vi "canDataSort.vi"() -> ()   [LabVIEW 2023] (continued)
16\t39\t88\r\n      2202  1FFFFFFF   00000004    8        00\t00\tFF\tFF\tFF\tFF\tFF\tFF\r\n      2193  18F106A7   00000004    8        00\tF7\tFF\tFF\tFF\tFF\tFF\t9C\r\n      2192  1FFFFFFF   00000004    8        00\t00\tFF\tFF\tFF\tFF\tFF\tFF\r\n      2183  0CF102A7   00000004    8        30\t75\tE0\t2E\t80\tFF\tFF\tFD\r\n      2183  0CF101A7   00000004    8        68\t00\t97\tCC\t00\t16\t39\t87\r\n      2182  1FFFFFFF   00000004    8        00\t00\tFF\tFF\tFF\tFF\tFF\tFF\r\n      2172  1FFFFFFF   00000004    8        00\t00\tFF\tFF\tFF\tFF\tFF\tFF\r\n      2223  0CF101A7   00000004    8        68\t00\t97\tCC\t00\t16\t39\t89\r\n      2222  1FFFFFFF   00000004    8        00\t00\tFF\tFF\tFF\tFF\tFF\tFF\r\n      2212  1FFFFFFF   00000004    8        00\t20\tFF\tFF\tFF\tFF\tFF\tFF\r\n      2203  0CF102A7   00000004    8        30\t75\tE0\t2E\t80\tFF\tFF\tFD\r\n      2203  0CF101A7   00000004    8        68\t00\t97\tCC\t00\t16\t39\t88\r\n      2202  1FFFFFFF   00000004    8        00\t00\tFF\tFF\tFF\tFF\tFF\tFF\r\n      2193  18F106A7   00000004    8        00\tF7\tFF\tFF\tFF\tFF\tFF\t9C\r\n      2192  1FFFFFFF   00000004    8        00\t00\tFF\tFF\tFF\tFF\tFF\tFF\r\n      2183  0CF102A7   00000004    8        30\t75\tE0\t2E\t80\tFF\tFF\tFD\r\n      2183  0CF101A7   00000004    8        68\t00\t97\tCC\t00\t16\t39\t87\r\n      2182  1FFFFFFF   00000004    8        00\t00\tFF\tFF\tFF\tFF\tFF\tFF\r\n      2223  0CF102A7   00000004    8        30\t75\tE0\t2E\t80\tFF\tFF\tFD\r\n      2223  0CF101A7   00000004    8        68\t00\t97\tCC\t00\t16\t39\t89\r\n      2222  1FFFFFFF   00000004    8        00\t00\tFF\tFF\tFF\tFF\tFF\tFF\r\n      2212  1FFFFFFF   00000004    8        00\t20\tFF\tFF\tFF\tFF\tFF\tFF\r\n      2203  0CF102A7   00000004    8        30\t75\tE0\t2E\t80\tFF\tFF\tFD\r\n      2203  0CF101A7   00000004    8        68\t00\t97\tCC\t00\t16\t39\t88\r\n      2202  1FFFFFFF   00000004    8        00\t00\tFF\tFF\tFF\tFF\tFF\tFF\r\n      2193  18F106A7   00000004    8        00\tF7\tFF\tFF\tFF\tFF\tFF\t9C\r\n      2192  1FFFFFFF   00000004    8        00\t00\tFF\tFF\tFF\tFF\tFF\tFF\r\n      2183  0CF102A7   00000004    8        30\t75\tE0\t2E\t80\tFF\tFF\tFD\r\n      2183  0CF101A7   00000004    8        68\t00\t97\tCC\t00\t16\t39\t87\r\n      2232  1FFFFFFF   00000004    8        00\t00\tFF\tFF\tFF\tFF\tFF\tFF\r\n      2223  0CF102A7   00000004    8        30\t75\tE0\t2E\t80\tFF\tFF\tFD\r\n      2223  0CF101A7   00000004    8        68\t00\t97\tCC\t00\t16\t39\t89\r\n      2222  1FFFFFFF   00000004    8        00\t00\tFF\tFF\tFF\tFF\tFF\tFF\r\n      2212  1FFFFFFF   00000004    8        00\t20\tFF\tFF\tFF\tFF\tFF\tFF\r\n      2203  0CF102A7   00000004    8        30\t75\tE0\t2E\t80\tFF\tFF\tFD\r\n      2203  0CF101A7   00000004    8        68\t00\t97\tCC\t00\t16\t39\t88\r\n      2202  1FFFFFFF   00000004    8        00\t00\tFF\tFF\tFF\tFF\tFF\tFF\r\n      2193  18F106A7   00000004    8        00\tF7\tFF\tFF\tFF\tFF\tFF\t9C\r\n      2192  1FFFFFFF   00000004    8        00\t00\tFF\tFF\tFF\tFF\tFF\tFF\r\n      2183  0CF102A7   00000004    8        30\t75\tE0\t2E\t80\tFF\tFF\tFD\r\n      2241  18F11FF0   00000004    8        FF\t3F\t90\t68\t88\t1B\t10\tEC\r\n      2232  1FFFFFFF   00000004    8        00\t00\tFF\tFF\tFF\tFF\tFF\tFF\r\n      2223  0CF102A7   00000004    8        30\t75\tE0\t2E\t80\tFF\tFF\tFD\r\n      2223  0CF101A7   00000004    8        68\t00\t97\tCC\t00\t16\t39\t89\r\n      2222  1FFFFFFF   00000004    8        00\t00\tFF\tFF\tFF\tFF\tFF\tFF\r\n      2212  1FFFFFFF   00000004    8        00\t20\tFF\tFF\tFF\tFF\tFF\tFF\r\n      2203  0CF102A7   00000004    8        30\t75\tE0\t2E\t80\tFF\tFF\tFD\r\n      2203  0CF101A7   00000004    8        68\t00\t97\tCC\t00\t16\t39\t88\r\n      2202  1FFFFFFF   00000004    8        00\t00\tFF\tFF\tFF\tFF\tFF\tFF\r\n      2193  18F106A7   00000004    8        00\tF7\tFF\tFF\tFF\tFF\tFF\t9C\r\n      2192  1FFFFFFF   00000004    8        00\t00\tFF\tFF\tFF\tFF\tFF\tFF\r\n      2242  18F120F0   00000004    8        2B\t75\t60\tB1\tB0\t01\tFF\tFF\r\n      2241  18F11FF0   00000004    8        FF\t3F\t90\t68\t88\t1B\t10\tEC\r\n      2232  1FFFFFFF   00000004    8        00\t00\tFF\tFF\tFF\tFF\tFF\tFF\r\n      2223  0CF102A7   00000004    8        30\t75\tE0\t2E\t80\tFF\tFF\tFD\r\n      2223  0CF101A7   00000004    8        68\t00\t97\tCC\t00\t16\t39\t89\r\n      2222  1FFFFFFF   00000004    8        00\t00\tFF\tFF\tFF\tFF\tFF\tFF\r\n      2212  1FFFFFFF   00000004    8        00\t20\tFF\tFF\tFF\tFF\tFF\tFF\r\n      2203  0CF102A7   00000004    8        30\t75\tE0\t2E\t80\tFF\tFF\tFD\r\n      2203  0CF101A7   00000004    8        68\t00\t97\tCC\t00\t16\t39\t88\r\n      2202  1FFFFFFF   00000004    8        00\t00\tFF\tFF\tFF\tFF\tFF\tFF\r\n      2193  18F106A7   00000004    8        00\tF7\tFF\tFF\tFF\tFF\tFF\t9C\r\n      2243  0CF101A7   00000004    8        68\t00\t97\tCC\t00\t16\t39\t8A\r\n      2242  18F120F0   00000004    8        2B\t75\t60\tB1\tB0\t01\tFF\tFF\r\n      2241  18F11FF0   00000004    8        FF\t3F\t90\t68\t88\t1B\t10\tEC\r\n      2232  1FFFFFFF   00000004    8        00\t00\tFF\tFF\tFF\tFF\tFF\tFF\r\n      2223  0CF102A7   00000004    8        30\t75\tE0\t2E\t80\tFF\tFF\tFD\r\n      2223  0CF101A7   00000004    8        68\t00\t97\tCC\t00\t16\t39\t89\r\n      2222  1FFFFFFF   00000004    8        00\t00\tFF\tFF\tFF\tFF\tFF\tFF\r\n      2212  1FFFFFFF   00000004    8        00\t20\tFF\tFF\tFF\tFF\tFF\tFF\r\n      2203  0CF102A7   00000004    8        30\t75\tE0\t2E\t80\tFF\tFF\tFD\r\n      2203  0CF101A7   00000004    8        68\t00\t97\tCC\t00\t16\t39\t88\r\n      2202  1FFFFFFF   00000004    8        00\t00\tFF\tFF\tFF\tFF\tFF\tFF\r\n      2243  0C3C4D4A   00000004    8        BE\tFF\tFF\t7F\t18\tFF\tFF\t4E\r\n      2243  0CF101A7   00000004    8        68\t00\t97\tCC\t00\t16\t39\t8A\r\n      2242  18F120F0   00000004    8        2B\t75\t60\tB1\tB0\t01\tFF\tFF\r\n      2241  18F11FF0   00000004    8        FF\t3F\t90\t68\t88\t1B\t10\tEC\r\n      2232  1FFFFFFF   00000004    8        00\t00\tFF\tFF\tFF\tFF\tFF\tFF\r\n      2223  0CF102A7   00000004    8        30\t75\tE0\t2E\t80\tFF\tFF\tFD\r\n      2223  0CF101A7   00000004    8        68\t00\t97\tCC\t00\t16\t39\t89\r\n      2222  1FFFFFFF   00000004    8        00\t00\tFF\tFF\tFF\tFF\tFF\tFF\r\n      2212  1FFFFFFF   00000004    8        00\t20\tFF\tFF\tFF\tFF\tFF\tFF\r\n      2203  0CF102A7   00000004    8        30\t75\tE0\t2E\t80\tFF\tFF\tFD\r\n      2203  0CF101A7   00000004    8        68\t00\t97\tCC\t00\t16\t39\t88\r\n      2244  0CF102A7   00000004    8        30\t75\tE0\t2E\t80\tFF\tFF\tFD\r\n      2243  0C3C4D4A   00000004    8        BE\tFF\tFF\t7F\t18\tFF\tFF\t4E\r\n      2243  0CF101A7   00000004    8        68\t00\t97\tCC\t00\t16\t39\t8A\r\n      2242  18F120F0   00000004    8        2B\t75\t60\tB1\tB0\t01\tFF\tFF\r\n      2241  18F11FF0   00000004    8        FF\t3F\t90\t68\t88\t1B\t10\tEC\r\n      2232  1FFFFFFF   00000004    8        00\t00\tFF\tFF\tFF\tFF\tFF\tFF\r\n      2223  0CF102A7   00000004    8        30\t75\tE0\t2E\t80\tFF\tFF\tFD\r\n      2223  0CF101A7   00000004    8        68\t00\t97\tCC\t00\t16\t39\t89\r\n      2222  1FFFFFFF   00000004    8        00\t00\tFF\tFF\tFF\tFF\tFF\tFF\r\n      2212  1FFFFFFF   00000004    8        00\t20\tFF\tFF\tFF\tFF\tFF\tFF\r\n      2203  0CF102A7   00000004    8        30\t75\tE0\t2E\t80\tFF\tFF\tFD\r\n      2244  0CF103A7   00000004    8        17\t1F\t08\t60\tB1\t1F\t08\t4E\r\n      2244  0CF102A7   00000004    8        30\t75\tE0\t2E\t80\tFF\tFF\tFD\r\n      2243  0C3C4D4A   00000004    8        BE\tFF\tFF\t7F\t18\tFF\tFF\t4E\r\n      2243  0CF101A7   00000004    8        68\t00\t97\tCC\t00\t16\t39\t8A\r\n      2242  18F120F0   00000004    8        2B\t75\t60\tB1\tB0\t01\tFF\tFF\r\n      2241  18F11FF0   00000004    8        FF\t3F\t90\t68\t88\t1B\t10\tEC\r\n      2232  1FFFFFFF   00000004    8        00\t00\tFF\tFF\tFF\tFF\tFF\tFF\r\n      2223  0CF102A7   00000004    8        30\t75\tE0\t2E\t80\tFF\tFF\tFD\r\n      2223  0CF101A7   00000004    8        68\t00\t97\tCC\t00\t16\t39\t89\r\n      2222  1FFFFFFF   00000004    8        00\t00\tFF\tFF\tFF\tFF\tFF\tFF\r\n      2212  1FFFFFFF   00000004    8        00\t20\tFF\tFF\tFF\tFF\tFF\tFF\r\n      2245  0CF104A7   00000004    8        F0\t60\t22\tFC\tFF\tFF\tFF\t4E\r\n      2244  0CF103A7   00000004    8        17\t1F\t08\t60\tB1\t1F\t08\t4E\r\n      2244  0CF102A7   00000004    8        30\t75\tE0\t2E\t80\tFF\tFF\tFD\r\n      2243  0C3C4D4A   00000004    8        BE\tFF\tFF\t7F\t18\tFF\tFF\t4E\r\n      2243  0CF101A7   00000004    8        68\t00\t97\tCC\t00\t16\t39\t8A\r\n      2242  18F120F0   00000004    8        2B\t75\t60\tB1\tB0\t01\tFF\tFF\r\n      2241  18F11FF0   00000004    8        FF\t3F\t90\t68\t88\t1B\t10\tEC\r\n      2232  1FFFFFFF   00000004    8        00\t00\tFF\tFF\tFF\tFF\tFF\tFF\r\n      2223  0CF102A7   00000004    8        30\t75\tE0\t2E\t80\tFF\tFF\tFD\r\n      2223  0CF101A7   00000004    8        68\t00\t97\tCC\t00\t16\t39\t89\r\n      2222  1FFFFFFF   00000004    8        00\t00\tFF\tFF\tFF\tFF\tFF\tFF\r\n      2245  18F106A7   00000004    8        00\tF7\tFF\tFF\tFF\tFF\tFF\t9D\r\n      2245  0CF104A7   00000004    8        F0\t60\t22\tFC\tFF\tFF\tFF\t4E\r\n      2244  0CF103A7   00000004    8        17\t1F\t08\t60\tB1\t1F\t08\t4E\r\n      2244  0CF102A7   00000004    8        30\t75\tE0\t2E\t80\tFF\tFF\tFD\r\n      2243  0C3C4D4A   00000004    8        BE\tFF\tFF\t7F\t18\tFF\tFF\t4E\r\n      2243  0CF101A7   00000004    8        68\t00\t97\tCC\t00\t16\t39\t8A\r\n      2242  18F120F0   00000004    8        2B\t75\t60\tB1\tB0\t01\tFF\tFF\r\n      2241  18F11FF0   00000004    8        FF\t3F\t90\t68\t88\t1B\t10\tEC\r\n      2232  1FFFFFFF   00000004    8        00\t00\tFF\tFF\tFF\tFF\tFF\tFF\r\n      2223  0CF102A7   00000004    8        30\t75\tE0\t2E\t80\tFF\tFF\tFD\r\n      2223  0CF101A7   00000004    8        68\t00\t97\tCC\t00\t16\t39\t89\r\n      2246  18F121F0   00000004    8        09\t19\t00\t00\tFF\tFF\tB0\t01\r\n      2245  18F106A7   00000004    8        00\tF7\tFF\tFF\tFF\tFF\tFF\t9D\r\n      2245  0CF104A7   00000004    8        F0\t60\t22\tFC\tFF\tFF\tFF\t4E\r\n      2244  0CF103A7   00000004    8        17\t1F\t08\t60\tB1\t1F\t08\t4E\r\n      2244  0CF102A7   00000004    8        30\t75\tE0\t2E\t80\tFF\tFF\tFD\r\n      2243  0C3C4D4A   00000004    8        BE\tFF\tFF\t7F\t18\tFF\tFF\t4E\r\n      2243  0CF101A7   00000004    8        68\t00\t97\tCC\t00\t16\t39\t8A\r\n      2242  18F120F0   00000004    8        2B\t75\t60\tB1\tB0\t01\tFF\tFF\r\n      2241  18F11FF0   00000004    8        FF\t3F\t90\t68\t88\t1B\t10\tEC\r\n      2232  1FFFFFFF   00000004    8        00\t00\tFF\tFF\tFF\tFF\tFF\tFF\r\n      2223  0CF102A7   00000004    8        30\t75\tE0\t2E\t80\tFF\tFF\tFD\r\n      2247  1FFFFFFF   00000004    8        00\t00\tFF\tFF\tFF\tFF\tFF\tFF\r\n      2246  18F121F0   00000004    8        09\t19\t00\t00\tFF\tFF\tB0\t01\r\n      2245  18F106A7   00000004    8        00\tF7\tFF\tFF\tFF\tFF\tFF\t9D\r\n      2245  0CF104A7   00000004    8        F0\t60\t22\tFC\tFF\tFF\tFF\t4E\r\n      2244  0CF103A7   00000004    8        17\t1F\t08\t60\tB1\t1F\t08\t4E\r\n      2244  0CF102A7   00000004    8        30\t75\tE0\t2E\t80\tFF\tFF\tFD\r\n      2243  0C3C4D4A   00000004    8        BE\tFF\tFF\t7F\t18\tFF\tFF\t4E\r\n      2243  0CF101A7   00000004    8        68\t00\t97\tCC\t00\t16\t39\t8A\r\n      2242  18F120F0   00000004    8        2B\t75\t60\tB1\tB0\t01\tFF\tFF\r\n      2241  18F11FF0   00000004    8        FF\t3F\t90\t68\t88\t1B\t10\tEC\r\n      2232  1FFFFFFF   00000004    8        00\t00\tFF\tFF\tFF\tFF\tFF\tFF\r\n      2252  1FFFFFFF   00000004    8        00\t20\tFF\tFF\tFF\tFF\tFF\tFF\r\n      2247  1FFFFFFF   00000004    8        00\t00\tFF\tFF\tFF\tFF\tFF\tFF\r\n      2246  18F121F0   00000004    8        09\t19\t00\t00\tFF\tFF\tB0\t01\r\n      2245  18F106A7   00000004    8        00\tF7\tFF\tFF\tFF\tFF\tFF\t9D\r\n      2245  0CF104A7   00000004    8        F0\t60\t22\tFC\tFF\tFF\tFF\t4E\r\n      2244  0CF103A7   00000004    8        17\t1F\t08\t60\tB1\t1F\t08\t4E\r\n      2244  0CF102A7   00000004    8        30\t75\tE0\t2E\t80\tFF\tFF\tFD\r\n      2243  0C3C4D4A   00000004    8        BE\tFF\tFF\t7F\t18\tFF\tFF\t4E\r\n      2243  0CF101A7   00000004    8        68\t00\t97\tCC\t00\t16\t39\t8A\r\n      2242  18F120F0   00000004    8        2B\t75\t60\tB1\tB0\t01\tFF\tFF\r\n      2241  18F11FF0   00000004    8        FF\t3F\t90\t68\t88\t1B\t10\tEC\r\n      2262  1FFFFFFF   00000004    8        00\t00\tFF\tFF\tFF\tFF\tFF\tFF\r\n      2252  1FFFFFFF   00000004    8        00\t20\tFF\tFF\tFF\tFF\tFF\tFF\r\n      2247  1FFFFFFF   00000004    8        00\t00\tFF\tFF\tFF\tFF\tFF\tFF\r\n      2246  18F121F0   00000004    8        09\t19\t00\t00\tFF\tFF\tB0\t01\r\n      2245  18F106A7   00000004    8        00\tF7\tFF\tFF\tFF\tFF\tFF\t9D\r\n      2245  0CF104A7   00000004    8        F0\t60\t22\tFC\tFF\tFF\tFF\t4E\r\n      2244  0CF103A7   00000004    8        17\t1F\t08\t60\tB1\t1F\t08\t4E\r\n      2244  0CF102A7   00000004    8        30\t75\tE0\t2E\t80\tFF\tFF\tFD\r\n      2243  0C3C4D4A   00000004    8        BE\tFF\tFF\t7F\t18\tFF\tFF\t4E\r\n      2243  0CF101A7   00000004    8        68\t00\t97\tCC\t00\t16\t39\t8A\r\n      2242  18F120F0   00000004    8        2B\t75\t60\tB1\tB0\t01\tFF\tFF\r\n      2263  0CF101A7   00000004    8        68\t00\t97\tCC\t00\t16\t39\t8B\r\n      2262  1FFFFFFF   00000004    8        00\t00\tFF\tFF\tFF\tFF\tFF\tFF\r\n      2252  1FFFFFFF   00000004    8        00\t20\tFF\tFF\tFF\tFF\tFF\tFF\r\n      2247  1FFFFFFF   00000004    8        00\t00\tFF\tFF\tFF\tFF\tFF\tFF\r\n      2246  18F121F0   00000004    8        09\t19\t00\t00\tFF\tFF\tB0\t01\r\n      2245  18F106A7   00000004    8        00\tF7\tFF\tFF\tFF\tFF\tFF\t9D\r\n      2245  0CF104A7   00000004    8        F0\t60\t22\tFC\tFF\tFF\tFF\t4E\r\n      2244  0CF103A7   00000004    8        17\t1F\t08\t60\tB1\t1F\t08\t4E\r\n      2244  0CF102A7   00000004    8        30\t75\tE0\t2E\t80\tFF\tFF\tFD\r\n      2243  0C3C4D4A   00000004    8        BE\tFF\tFF\t7F\t18\tFF\tFF\t4E\r\n      2243  0CF101A7   00000004    8        68\t00\t97\tCC\t00\t16\t39\t8A\r\n      2263  0CF102A7   00000004    8        30\t75\tE0\t2E\t80\tFF\tFF\tFD\r\n      2263  0CF101A7   00000004    8        68\t00\t97\tCC\t00\t16\t39\t8B\r\n      2262  1FFFFFFF   00000004    8        00\t00\tFF\tFF\tFF\tFF\tFF\tFF\r\n      2252  1FFFFFFF   00000004    8        00\t20\tFF\tFF\tFF\tFF\tFF\tFF\r\n      2247  1FFFFFFF   00000004    8        00\t00\tFF\tFF\tFF\tFF\tFF\tFF\r\n      2246  18F121F0   00000004    8        09\t19\t00\t00\tFF\tFF\tB0\t01\r\n      2245  18F106A7   00000004    8        00\tF7\tFF\tFF\tFF\tFF\tFF\t9D\r\n      2245  0CF104A7   00000004    8        F0\t60\t22\tFC\tFF\tFF\tFF\t4E\r\n      2244  0CF103A7   00000004    8        17\t1F\t08\t60\tB1\t1F\t08\t4E\r\n      2244  0CF102A7   00000004    8        30\t75\tE0\t2E\t80\tFF\tFF\tFD\r\n      2243  0C3C4D4A   00000004    8        BE\tFF\tFF\t7F\t18\tFF\tFF\t4E\r\n      2272  1FFFFFFF   00000004    8        00\t20\tFF\tFF\tFF\tFF\tFF\tFF\r\n      2263  0CF102A7   00000004    8        30\t75\tE0\t2E\t80\tFF\tFF\tFD\r\n      2263  0CF101A7   00000004    8        68\t00\t97\tCC\t00\t16\t39\t8B\r\n      2262  1FFFFFFF   00000004    8        00\t00\tFF\tFF\tFF\tFF\tFF\tFF\r\n      2252  1FFFFFFF   00000004    8        00\t20\tFF\tFF\tFF\tFF\tFF\tFF\r\n      2247  1FFFFFFF   00000004    8        00\t00\tFF\tFF\tFF\tFF\tFF\tFF\r\n      2246  18F121F0   00000004    8        09\t19\t00\t00\tFF\tFF\tB0\t01\r\n      2245  18F106A7   00000004    8        00\tF7\tFF\tFF\tFF\tFF\tFF\t9D\r\n      2245  0CF104A7   00000004    8        F0\t60\t22\tFC\tFF\tFF\tFF\t4E\r\n      2244  0CF103A7   00000004    8        17\t1F\t08\t60\tB1\t1F\t08\t4E\r\n      2244  0CF102A7   00000004    8        30\t75\tE0\t2E\t80\tFF\tFF\tFD\r\n      2282  1FFFFFFF   00000004    8        00\t20\tFF\tFF\tFF\tFF\tFF\tFF\r\n      2272  1FFFFFFF   00000004    8        00\t20\tFF\tFF\tFF\tFF\tFF\tFF\r\n      2263  0CF102A7   00000004    8        30\t75\tE0\t2E\t80\tFF\tFF\tFD\r\n      2263  0CF101A7   00000004    8        68\t00\t97\tCC\t00\t16\t39\t8B\r\n      2262  1FFFFFFF   00000004    8        00\t00\tFF\tFF\tFF\tFF\tFF\tFF\r\n      2252  1FFFFFFF   00000004    8        00\t20\tFF\tFF\tFF\tFF\tFF\tFF\r\n      2247  1FFFFFFF   00000004    8        00\t00\tFF\tFF\tFF\tFF\tFF\tFF\r\n      2246  18F121F0   00000004    8        09\t19\t00\t00\tFF\tFF\tB0\t01\r\n      2245  18F106A7   00000004    8        00\tF7\tFF\tFF\tFF\tFF\tFF\t9D\r\n      2245  0CF104A7   00000004    8        F0\t60\t22\tFC\tFF\tFF\tFF\t4E\r\n      2244  0CF103A7   00000004    8        17\t1F\t08\t60\tB1\t1F\t08\t4E\r\n      2283  0CF101A7   00000004    8        68\t00\t97\tCC\t00\t16\t39\t8C\r\n      2282  1FFFFFFF   00000004    8        00\t20\tFF\tFF\tFF\tFF\tFF\tFF\r\n      2272  1FFFFFFF   00000004    8        00\t20\tFF\tFF\tFF\tFF\tFF\tFF\r\n      2263  0CF102A7   00000004    8        30\t75\tE0\t2E\t80\tFF\tFF\tFD\r\n      2263  0CF101A7   00000004    8        68\t00\t97\tCC\t00\t16\t39\t8B\r\n      2262  1FFFFFFF   00000004    8        00\t00\tFF\tFF\tFF\tFF\tFF\tFF\r\n      2252  1FFFFFFF   00000004    8        00\t20\tFF\tFF\tFF\tFF\tFF\tFF\r\n      2247  1FFFFFFF   00000004    8        00\t00\tFF\tFF\tFF\tFF\tFF\tFF\r\n      2246  18F121F0   00000004    8        09\t19\t00\t00\tFF\tFF\tB0\t01\r\n      2245  18F106A7   00000004    8        00\tF7\tFF\tFF\tFF\tFF\tFF\t9D\r\n      2245  0CF104A7   00000004    8        F0\t60\t22\tFC\tFF\tFF\tFF\t4E\r\n      2283  0CF102A7   00000004    8        30\t75\tE0\t2E\t80\tFF\tFF\tFD\r\n      2283  0CF101A7   00000004    8        68\t00\t97\tCC\t00\t16\t39\t8C\r\n      2282  1FFFFFFF   00000004    8        00\t20\tFF\tFF\tFF\tFF\tFF\tFF\r\n      2272  1FFFFFFF   00000004    8        00\t20\tFF\tFF\tFF\tFF\tFF\tFF\r\n      2263  0CF102A7   00000004    8        30\t75\tE0\t2E\t80\tFF\tFF\tFD\r\n      2263  0CF101A7   00000004    8        68\t00\t97\tCC\t00\t16\t39\t8B\r\n      2262  1FFFFFFF   00000004    8        00\t00\tFF\tFF\tFF\tFF\tFF\tFF\r\n      2252  1FFFFFFF   00000004    8        00\t20\tFF\tFF\tFF\tFF\tFF\tFF\r\n      2247  1FFFFFFF   00000004    8        00\t00\tFF\tFF\tFF\tFF\tFF\tFF\r\n      2246  18F121F0   00000004    8        09\t19\t00\t00\tFF\tFF\tB0\t01\r\n      2245  18F106A7   00000004    8        00\tF7\tFF\tFF\tFF\tFF\tFF\t9D\r\n      2292  1FFFFFFF   00000004    8        00\t20\tFF\tFF\tFF\tFF\tFF\tFF\r\n      2283  0CF102A7   00000004    8        30\t75\tE0\t2E\t80\tFF\tFF\tFD\r\n      2283  0CF101A7   00000004    8        68\t00\t97\tCC\t00\t16\t39\t8C\r\n      2282  1FFFFFFF   00000004    8        00\t20\tFF\tFF\tFF\tFF\tFF\tFF\r\n      2272  1FFFFFFF   00000004    8        00\t20\tFF\tFF\tFF\tFF\tFF\tFF\r\n      2263  0CF102A7   00000004    8        30\t75\tE0\t2E\t80\tFF\tFF\tFD\r\n      2263  0CF101A7   00000004    8        68\t00\t97\tCC\t00\t16\t39\t8B\r\n      2262  1FFFFFFF   00000004    8        00\t00\tFF\tFF\tFF\tFF\tFF\tFF\r\n      2252  1FFFFFFF   00000004    8        00\t20\tFF\tFF\tFF\tFF\tFF\tFF\r\n      2247  1FFFFFFF   00000004    8        00\t00\tFF\tFF\tFF\tFF\tFF\tFF\r\n      2246  18F121F0   00000004    8        09\t19\t00\t00\tFF\tFF\tB0\t01\r\n      2293  18F106A7   00000004    8        00\tF7\tFF\tFF\tFF\tFF\tFF\t9E\r\n      2292  1FFFFFFF   00000004    8        00\t20\tFF\tFF\tFF\tFF\tFF\tFF\r\n      2283  0CF102A7   00000004    8        30\t75\tE0\t2E\t80\tFF\tFF\tFD\r\n      2283  0CF101A7   00000004    8        68\t00\t97\tCC\t00\t16\t39\t8C\r\n      2282  1FFFFFFF   00000004    8        00\t20\tFF\tFF\tFF\tFF\tFF\tFF\r\n      2272  1FFFFFFF   00000004    8        00\t20\tFF\tFF\tFF\tFF\tFF\tFF\r\n      2263  0CF102A7   00000004    8        30\t75\tE0\t2E\t80\tFF\tFF\tFD\r\n      2263  0CF101A7   00000004    8        68\t00\t97\tCC\t00\t16\t39\t8B\r\n      2262  1FFFFFFF   00000004    8        00\t00\tFF\tFF\tFF\tFF\tFF\tFF\r\n      2252  1FFFFFFF   00000004    8        00\t20\tFF\tFF\tFF\tFF\tFF\tFF\r\n      2247  1FFFFFFF   00000004    8        00\t00\tFF\tFF\tFF\tFF\tFF\tFF\r\n      2302  1FFFFFFF   00000004    8        00\t00\tFF\tFF\tFF\tFF\tFF\tFF\r\n      2293  18F106A7   00000004    8        00\tF7\tFF\tFF\tFF\tFF\tFF\t9E\r\n      2292  1FFFFFFF   00000004    8        00\t20\tFF\tFF\tFF\tFF\tFF\tFF\r\n      2283  0CF102A7   00000004    8        30\t75\tE0\t2E\t80\tFF\tFF\tFD\r\n      2283  0CF101A7   00000004    8        68\t00\t97\tCC\t00\t16\t39\t8C\r\n      2282  1FFFFFFF   00000004    8        00\t20\tFF\tFF\tFF\tFF\tFF\tFF\r\n      2272  1FFFFFFF   00000004    8        00\t20\tFF\tFF\tFF\tFF\tFF\tFF\r\n      2263  0CF102A7   00000004    8        30\t75\tE0\t2E\t80\tFF\tFF\tFD\r\n      2263  0CF101A7   00000004    8        68\t00\t97\tCC\t00\t16\t39\t8B\r\n      2262  1FFFFFFF   00000004    8        00\t00\tFF\tFF\tFF\tFF\tFF\tFF\r\n      2252  1FFFFFFF   00000004    8        00\t20\tFF\tFF\tFF\tFF\tFF\tFF\r\n      2303  0CF101A7   00000004    8        68\t00\t97\tCC\t00\t16\t39\t8D\r\n      2302  1FFFFFFF   00000004    8        00\t00\tFF\tFF\tFF\tFF\tFF\tFF\r\n      2293  18F106A7   00000004    8        00\tF7\tFF\tFF\tFF\tFF\tFF\t9E\r\n      2292  1FFFFFFF   00000004    8        00\t20\tFF\tFF\tFF\tFF\tFF\tFF\r\n      2283  0CF102A7   00000004    8        30\t75\tE0\t2E\t80\tFF\tFF\tFD\r\n      2283  0CF101A7   00000004    8        68\t00\t97\tCC\t00\t16\t39\t8C\r\n      2282  1FFFFFFF   00000004    8        00\t20\tFF\tFF\tFF\tFF\tFF\tFF\r\n      2272  1FFFFFFF   00000004    8        00\t20\tFF\tFF\tFF\tFF\tFF\tFF\r\n      2263  0CF102A7   00000004    8        30\t75\tE0\t2E\t80\tFF\tFF\tFD\r\n      2263  0CF101A7   00000004    8        68\t00\t97\tCC\t00\t16\t39\t8B\r\n      2262  1FFFFFFF   00000004    8        00\t00\tFF\tFF\tFF\tFF\tFF\tFF\r\n      2303  0CF102A7   00000004    8        30\t75\tE0\t2E\t80\tFF\tFF\tFD\r\n      2303  0CF101A7   00000004    8        68\t00\t97\tCC\t00\t16\t39\t8D\r\n      2302  1FFFFFFF   00000004    8        00\t00\tFF\tFF\tFF\tFF\tFF\tFF\r\n      2293  18F106A7   00000004    8        00\tF7\tFF\tFF\tFF\tFF\tFF\t9E\r\n      2292  1FFFFFFF   00000004    8        00\t20\tFF\tFF\tFF\tFF\tFF\tFF\r\n      2283  0CF102A7   00000004    8        30\t75\tE0\t2E\t80\tFF\tFF\tFD\r\n      2283  0CF101A7   00000004    8        68\t00\t97\tCC\t00\t16\t39\t8C\r\n      2282  1FFFFFFF   00000004    8        00\t20\tFF\tFF\tFF\tFF\tFF\tFF\r\n      2272  1FFFFFFF   00000004    8        00\t20\tFF\tFF\tFF\tFF\tFF\tFF\r\n      2263  0CF102A7   00000004    8        30\t75\tE0\t2E\t80\tFF\tFF\tFD\r\n      2263  0CF101A7   00000004    8        68\t00\t97\tCC\t00\t16\t39\t8B\r\n      2312  1FFFFFFF   00000004    8        00\t20\tFF\tFF\tFF\tFF\tFF\tFF\r\n      2303  0CF102A7   00000004    8        30\t75\tE0\t2E\t80\tFF\tFF\tFD\r\n      2303  0CF101A7   00000004    8        68\t00\t97\tCC\t00\t16\t39\t8D\r\n      2302  1FFFFFFF   00000004    8        00\t00\tFF\tFF\tFF\tFF\tFF\tFF\r\n      2293  18F106A7   00000004    8        00\tF7\tFF\tFF\tFF\tFF\tFF\t9E\r\n      2292  1FFFFFFF   00000004    8        00\t20\tFF\tFF\tFF\tFF\tFF\tFF\r\n      2283  0CF102A7   00000004    8        30\t75\tE0\t2E\t80\tFF\tFF\tFD\r\n      2283  0CF101A7   00000004    8        68\t00\t97\tCC\t00\t16\t39\t8C\r\n      2282  1FFFFFFF   00000004    8        00\t20\tFF\tFF\tFF\tFF\tFF\tFF\r\n      2272  1FFFFFFF   00000004    8        00\t20\tFF\tFF\tFF\tFF\tFF\tFF\r\n      2263  0CF102A7   00000004    8        30\t75\tE0\t2E\t80\tFF\tFF\tFD\r\n      2322  1FFFFFFF   00000004    8        00\t00\tFF\tFF\tFF\tFF\tFF\tFF\r\n      2312  1FFFFFFF   00000004    8        00\t20\tFF\tFF\tFF\tFF\tFF\tFF\r\n      2303  0CF102A7   00000004    8        30\t75\tE0\t2E\t80\tFF\tFF\tFD\r\n      2303  0CF101A7   00000004    8        68\t00\t97\tCC\t00\t16\t39\t8D\r\n      2302  1FFFFFFF   00000004    8        00\t00\tFF\tFF\tFF\tFF\tFF\tFF\r\n      2293  18F106A7   00000004    8        00\tF7\tFF\tFF\tFF\tFF\tFF\t9E\r\n      2292  1FFFFFFF   00000004    8        00\t20\tFF\tFF\tFF\tFF\tFF\tFF\r\n      2283  0CF102A7   00000004    8        30\t75\tE0\t2E\t80\tFF\tFF\tFD\r\n      2283  0CF101A7   00000004    8        68\t00\t97\tCC\t00\t16\t39\t8C\r\n      2282  1FFFFFFF   00000004    8        00\t20\tFF\tFF\tFF\tFF\tFF\tFF\r\n      2272  1FFFFFFF   00000004    8        00\t20\tFF\tFF\tFF\tFF\tFF\tFF\r\n      2323  0CF101A7   00000004    8        68\t00\t97\tCC\t00\t16\t39\t8E\r\n      2322  1FFFFFFF   00000004    8        00\t00\tFF\tFF\tFF\tFF\tFF\tFF\r\n      2312  1FFFFFFF   00000004    8        00\t20\tFF\tFF\tFF\tFF\tFF\tFF\r\n      2303  0CF102A7   00000004    8        30\t75\tE0\t2E\t80\tFF\tFF\tFD\r\n      2303  0CF101A7   00000004    8        68\t00\t97\tCC\t00\t16\t39\t8D\r\n      2302  1FFFFFFF   00000004    8        00\t00\tFF\tFF\tFF\tFF\tFF\tFF\r\n      2293  18F106A7   00000004    8        00\tF7\tFF\tFF\tFF\tFF\tFF\t9E\r\n      2292  1FFFFFFF   00000004    8        00\t20\tFF\tFF\tFF\tFF\tFF\tFF\r\n      2283  0CF102A7   00000004    8        30\t75\tE0\t2E\t80\tFF\tFF\tFD\r\n      2283  0CF101A7   00000004    8        68\t00\t97\tCC\t00\t16\t39\t8C\r\n      2282  1FFFFFFF   00000004    8        00\t20\tFF\tFF\tFF\tFF\tFF\tFF\r\n      2323  0CF102A7   00000004    8        30\t75\tE0\t2E\t80\tFF\tFF\tFD\r\n      2323  0CF101A7   00000004    8        68\t00\t97\tCC\t00\t16\t39\t8E\r\n      2322  1FFFFFFF   00000004    8        00\t00\tFF\tFF\tFF\tFF\tFF\tFF\r\n      2312  1FFFFFFF   00000004    8        00\t20\tFF\tFF\tFF\tFF\tFF\tFF\r\n      2303  0CF102A7   00000004    8        30\t75\tE0\t2E\t80\tFF\tFF\tFD\r\n      2303  0CF101A7   00000004    8        68\t00\t97\tCC\t00\t16\t39\t8D\r\n      2302  1FFFFFFF   00000004    8        00\t00\tFF\tFF\tFF\tFF\tFF\tFF\r\n      2293  18F106A7   00000004    8        00\tF7\tFF\tFF\tFF\tFF\tFF\t9E\r\n      2292  1FFFFFFF   00000004    8        00\t20\tFF\tFF\tFF\tFF\tFF\tFF\r\n      2283  0CF102A7   00000004    8        30\t75\tE0\t2E\t80\tFF\tFF\tFD\r\n      2283  0CF101A7   00000004    8        68\t00\t97\tCC\t00\t16\t39\t8C\r\n      2332  1FFFFFFF   00000004    8        00\t20\tFF\tFF\tFF\tFF\tFF\tFF\r\n      2323  0CF102A7   00000004    8        30\t75\tE0\t2E\t80\tFF\tFF\tFD\r\n      2323  0CF101A7   00000004    8        68\t00\t97\tCC\t00\t16\t39\t8E\r\n      2322  1FFFFFFF   00000004    8        00\t00\tFF\tFF\tFF\tFF\tFF\tFF\r\n      2312  1FFFFFFF   00000004    8        00\t20\tFF\tFF\tFF\tFF\tFF\tFF\r\n      2303  0CF102A7   00000004    8        30\t75\tE0\t2E\t80\tFF\tFF\tFD\r\n      2303  0CF101A7   00000004    8        68\t00\t97\tCC\t00\t16\t39\t8D\r\n      2302  1FFFFFFF   00000004    8        00\t00\tFF\tFF\tFF\tFF\tFF\tFF\r\n      2293  18F106A7   00000004    8        00\tF7\tFF\tFF\tFF\tFF\tFF\t9E\r\n      2292  1FFFFFFF   00000004    8        00\t20\tFF\tFF\tFF\tFF\tFF\tFF\r\n      2283  0CF102A7   00000004    8        30\t75\tE0\t2E\t80\tFF\tFF\tFD\r\n      2341  18F11FF0   00000004    8        FF\t3F\t90\t68\t88\t1B\t10\tFC\r\n      2332  1FFFFFFF   00000004    8        00\t20\tFF\tFF\tFF\tFF\tFF\tFF\r\n      2323  0CF102A7   00000004    8        30\t75\tE0\t2E\t80\tFF\tFF\tFD\r\n      2323  0CF101A7   00000004    8        68\t00\t97\tCC\t00\t16\t39\t8E\r\n      2322  1FFFFFFF   00000004    8        00\t00\tFF\tFF\tFF\tFF\tFF\tFF\r\n      2312  1FFFFFFF   00000004    8        00\t20\tFF\tFF\tFF\tFF\tFF\tFF\r\n      2303  0CF102A7   00000004    8        30\t75\tE0\t2E\t80\tFF\tFF\tFD\r\n      2303  0CF101A7   00000004    8        68\t00\t97\tCC\t00\t16\t39\t8D\r\n      2302  1FFFFFFF   00000004    8        00\t00\tFF\tFF\tFF\tFF\tFF\tFF\r\n      2293  18F106A7   00000004    8        00\tF7\tFF\tFF\tFF\tFF\tFF\t9E\r\n      2292  1FFFFFFF   00000004    8        00\t20\tFF\tFF\tFF\tFF\tFF\tFF\r\n      2342  18F120F0   00000004    8        2B\t75\t60\tB1\tB0\t01\tFF\tFF\r\n      2341  18F11FF0   00000004    8        FF\t3F\t90\t68\t88\t1B\t10\tFC\r\n      2332  1FFFFFFF   00000004    8        00\t20\tFF\tFF\tFF\tFF\tFF\tFF\r\n      2323  0CF102A7   00000004    8        30\t75\tE0\t2E\t80\tFF\tFF\tFD\r\n      2323  0CF101A7   00000004    8        68\t00\t97\tCC\t00\t16\t39\t8E\r\n      2322  1FFFFFFF   00000004    8        00\t00\tFF\tFF\tFF\tFF\tFF\tFF\r\n      2312  1FFFFFFF   00000004    8        00\t20\tFF\tFF\tFF\tFF\tFF\tFF\r\n      2303  0CF102A7   00000004    8        30\t75\tE0\t2E\t80\tFF\tFF\tFD\r\n      2303  0CF101A7   00000004    8        68\t00\t97\tCC\t00\t16\t39\t8D\r\n      2302  1FFFFFFF   00000004    8        00\t00\tFF\tFF\tFF\tFF\tFF\tFF\r\n      2293  18F106A7   00000004    8        00\tF7\tFF\tFF\tFF\tFF\tFF\t9E\r\n      2343  0CF101A7   00000004    8        68\t00\t97\tCC\t00\t16\t39\t8F\r\n      2342  18F120F0   00000004    8        2B\t75\t60\tB1\tB0\t01\tFF\tFF\r\n      2341  18F11FF0   00000004    8        FF\t3F\t90\t68\t88\t1B\t10\tFC\r\n      2332  1FFFFFFF   00000004    8        00\t20\tFF\tFF\tFF\tFF\tFF\tFF\r\n      2323  0CF102A7   00000004    8        30\t75\tE0\t2E\t80\tFF\tFF\tFD\r\n      2323  0CF101A7   00000004    8        68\t00\t97\tCC\t00\t16\t39\t8E\r\n      2322  1FFFFFFF   00000004    8        00\t00\tFF\tFF\tFF\tFF\tFF\tFF\r\n      2312  1FFFFFFF   00000004    8        00\t20\tFF\tFF\tFF\tFF\tFF\tFF\r\n      2303  0CF102A7   00000004    8        30\t75\tE0\t2E\t80\tFF\tFF\tFD\r\n      2303  0CF101A7   00000004    8        68\t00\t97\tCC\t00\t16\t39\t8D\r\n      2302  1FFFFFFF   00000004    8        00\t00\tFF\tFF\tFF\tFF\tFF\tFF\r\n      2343  0C3C4D4A   00000004    8        BE\tFF\tFF\t7F\t18\tFF\tFF\t4F\r\n      2343  0CF101A7   00000004    8        68\t00\t97\tCC\t00\t16\t39\t8F\r\n      2342  18F120F0   00000004    8        2B\t75\t60\tB1\tB0\t01\tFF\tFF\r\n      2341  18F11FF0   00000004    8        FF\t3F\t90\t68\t88\t1B\t10\tFC\r\n      2332  1FFFFFFF   00000004    8        00\t20\tFF\tFF\tFF\tFF\tFF\tFF\r\n      2323  0CF102A7   00000004    8        30\t75\tE0\t2E\t80\tFF\tFF\tFD\r\n      2323  0CF101A7   00000004    8        68\t00\t97\tCC\t00\t16\t39\t8E\r\n      2322  1FFFFFFF   00000004    8        00\t00\tFF\tFF\tFF\tFF\tFF\tFF\r\n      2312  1FFFFFFF   00000004    8        00\t20\tFF\tFF\tFF\tFF\tFF\tFF\r\n      2303  0CF102A7   00000004    8        30\t75\tE0\t2E\t80\tFF\tFF\tFD\r\n      2303  0CF101A7   00000004    8        68\t00\t97\tCC\t00\t16\t39\t8D\r\n      2344  0CF102A7   00000004    8        30\t75\tE0\t2E\t80\tFF\tFF\tFD\r\n      2343  0C3C4D4A   00000004    8        BE\tFF\tFF\t7F\t18\tFF\tFF\t4F\r\n      2343  0CF101A7   00000004    8        68\t00\t97\tCC\t00\t16\t39\t8F\r\n      2342  18F120F0   00000004    8        2B\t75\t60\tB1\tB0\t01\tFF\tFF\r\n      2341  18F11FF0   00000004    8        FF\t3F\t90\t68\t88\t1B\t10\tFC\r\n      2332  1FFFFFFF   00000004    8        00\t20\tFF\tFF\tFF\tFF\tFF\tFF\r\n      2323  0CF102A7   00000004    8        30\t75\tE0\t2E\t80\tFF\tFF\tFD\r\n      2323  0CF101A7   00000004    8        68\t00\t97\tCC\t00\t16\t39\t8E\r\n      2322  1FFFFFFF   00000004    8        00\t00\tFF\tFF\tFF\tFF\tFF\tFF\r\n      2312  1FFFFFFF   00000004    8        00\t20\tFF\tFF\tFF\tFF\tFF\tFF\r\n      2303  0CF102A7   00000004    8        30\t75\tE0\t2E\t80\tFF\tFF\tFD\r\n      2344  0CF103A7   00000004    8        17\t1F\t08\t60\tB1\t1F\t08\t4F\r\n      2344  0CF102A7   00000004    8        30\t75\tE0\t2E\t80\tFF\tFF\tFD\r\n      2343  0C3C4D4A   00000004    8        BE\tFF\tFF\t7F\t18\tFF\tFF\t4F\r\n      2343  0CF101A7   00000004    8        68\t00\t97\tCC\t00\t16\t39\t8F\r\n      2342  18F120F0   00000004    8        2B\t75\t60\tB1\tB0\t01\tFF\tFF\r\n      2341  18F11FF0   00000004    8        FF\t3F\t90\t68\t88\t1B\t10\tFC\r\n      2332  1FFFFFFF   00000004    8        00\t20\tFF\tFF\tFF\tFF\tFF\tFF\r\n      2323  0CF102A7   00000004    8        30\t75\tE0\t2E\t80\tFF\tFF\tFD\r\n      2323  0CF101A7   00000004    8        68\t00\t97\tCC\t00\t16\t39\t8E\r\n      2322  1FFFFFFF   00000004    8        00\t00\tFF\tFF\tFF\tFF\tFF\tFF\r\n      2312  1FFFFFFF   00000004    8        00\t20\tFF\tFF\tFF\tFF\tFF\tFF\r\n      2345  0CF104A7   00000004    8        F0\t60\t22\tFC\tFF\tFF\tFF\t4F\r\n      2344  0CF103A7   00000004    8        17\t1F\t08\t60\tB1\t1F\t08\t4F\r\n      2344  0CF102A7   00000004    8        30\t75\tE0\t2E\t80\tFF\tFF\tFD\r\n      2343  0C3C4D4A   00000004    8        BE\tFF\tFF\t7F\t18\tFF\tFF\t4F\r\n      2343  0CF101A7   00000004    8        68\t00\t97\tCC\t00\t16\t39\t8F\r\n      2342  18F120F0   00000004    8        2B\t75\t60\tB1\tB0\t01\tFF\tFF\r\n      2341  18F11FF0   00000004    8        FF\t3F\t90\t68\t88\t1B\t10\tFC\r\n      2332  1FFFFFFF   00000004    8        00\t20\tFF\tFF\tFF\tFF\tFF\tFF\r\n      2323  0CF102A7   00000004    8        30\t75\tE0\t2E\t80\tFF\tFF\tFD\r\n      2323  0CF101A7   00000004    8        68\t00\t97\tCC\t00\t16\t39\t8E\r\n      2322  1FFFFFFF   00000004    8        00\t00\tFF\tFF\tFF\tFF\tFF\tFF\r\n      2345  18F106A7   00000004    8        00\tF7\tFF\tFF\tFF\tFF\tFF\t9F\r\n      2345  0CF104A7   00000004    8        F0\t60\t22\tFC\tFF\tFF\tFF\t4F\r\n      2344  0CF103A7   00000004    8        17\t1F\t08\t60\tB1\t1F\t08\t4F\r\n      2344  0CF102A7   00000004    8        30\t75\tE0\t2E\t80\tFF\tFF\tFD\r\n      2343  0C3C4D4A   00000004    8        BE\tFF\tFF\t7F\t18\tFF\tFF\t4F\r\n      2343  0CF101A7   00000004    8        68\t00\t97\tCC\t00\t16\t39\t8F\r\n      2342  18F120F0   00000004    8        2B\t75\t60\tB1\tB0\t01\tFF\tFF\r\n      2341  18F11FF0   00000004    8        FF\t3F\t90\t68\t88\t1B\t10\tFC\r\n      2332  1FFFFFFF   00000004    8        00\t20\tFF\tFF\tFF\tFF\tFF\tFF\r\n      2323  0CF102A7   00000004    8        30\t75\tE0\t2E\t80\tFF\tFF\tFD\r\n      2323  0CF101A7   00000004    8        68\t00\t97\tCC\t00\t16\t39\t8E\r\n      2346  18F121F0   00000004    8        09\t19\t00\t00\tFF\tFF\tB0\t01\r\n      2345  18F106A7   00000004    8        00\tF7\tFF\tFF\tFF\tFF\tFF\t9F\r\n      2345  0CF104A7   00000004    8        F0\t60\t22\tFC\tFF\tFF\tFF\t4F\r\n      2344  0CF103A7   00000004    8        17\t1F\t08\t60\tB1\t1F\t08\t4F\r\n      2344  0CF102A7   00000004    8        30\t75\tE0\t2E\t80\tFF\tFF\tFD\r\n      2343  0C3C4D4A   00000004    8        BE\tFF\tFF\t7F\t18\tFF\tFF\t4F\r\n      2343  0CF101A7   00000004    8        68\t00\t97\tCC\t00\t16\t39\t8F\r\n      2342  18F120F0   00000004    8        2B\t75\t60\tB1\tB0\t01\tFF\tFF\r\n      2341  18F11FF0   00000004    8        FF\t3F\t90\t68\t88\t1B\t10\tFC\r\n      2332  1FFFFFFF   00000004    8        00\t20\tFF\tFF\tFF\tFF\tFF\tFF\r\n      2323  0CF102A7   00000004    8        30\t75\tE0\t2E\t80\tFF\tFF\tFD\r\n      2347  1FFFFFFF   00000004    8        00\t20\tFF\tFF\tFF\tFF\tFF\tFF\r\n      2346  18F121F0   00000004    8        09\t19\t00\t00\tFF\tFF\tB0\t01\r\n      2345  18F106A7   00000004    8        00\tF7\tFF\tFF\tFF\tFF\tFF\t9F\r\n      2345  0CF104A7   00000004    8        F0\t60\t22\tFC\tFF\tFF\tFF\t4F\r\n      2344  0CF103A7   00000004    8        17\t1F\t08\t60\tB1\t1F\t08\t4F\r\n      2344  0CF102A7   00000004    8        30\t75\tE0\t2E\t80\tFF\tFF\tFD\r\n      2343  0C3C4D4A   00000004    8        BE\tFF\tFF\t7F\t18\tFF\tFF\t4F\r\n      2343  0CF101A7   00000004    8        68\t00\t97\tCC\t00\t16\t39\t8F\r\n      2342  18F120F0   00000004    8        2B\t75\t60\tB1\tB0\t01\tFF\tFF\r\n      2341  18F11FF0   00000004    8        FF\t3F\t90\t68\t88\t1B\t10\tFC\r\n      2332  1FFFFFFF   00000004    8        00\t20\tFF\tFF\tFF\tFF\tFF\tFF\r\n      2352  1FFFFFFF   00000004    8        00\t20\tFF\tFF\tFF\tFF\tFF\tFF\r\n      2347  1FFFFFFF   00000004    8        00\t20\tFF\tFF\tFF\tFF\tFF\tFF\r\n      2346  18F121F0   00000004    8        09\t19\t00\t00\tFF\tFF\tB0\t01\r\n      2345  18F106A7   00000004    8        00\tF7\tFF\tFF\tFF\tFF\tFF\t9F\r\n      2345  0CF104A7   00000004    8        F0\t60\t22\tFC\tFF\tFF\tFF\t4F\r\n      2344  0CF103A7   00000004    8        17\t1F\t08\t60\tB1\t1F\t08\t4F\r\n      2344  0CF102A7   00000004    8        30\t75\tE0\t2E\t80\tFF\tFF\tFD\r\n      2343  0C3C4D4A   00000004    8        BE\tFF\tFF\t7F\t18\tFF\tFF\t4F\r\n      2343  0CF101A7   00000004    8        68\t00\t97\tCC\t00\t16\t39\t8F\r\n      2342  18F120F0   00000004    8        2B\t75\t60\tB1\tB0\t01\tFF\tFF\r\n      2341  18F11FF0   00000004    8        FF\t3F\t90\t68\t88\t1B\t10\tFC\r\n      2362  1FFFFFFF   00000004    8        00\t00\tFF\tFF\tFF\tFF\tFF\tFF\r\n      2352  1FFFFFFF   00000004    8        00\t20\tFF\tFF\tFF\tFF\tFF\tFF\r\n      2347  1FFFFFFF   00000004    8        00\t20\tFF\tFF\tFF\tFF\tFF\tFF\r\n      2346  18F121F0   00000004    8        09\t19\t00\t00\tFF\tFF\tB0\t01\r\n      2345  18F106A7   00000004    8        00\tF7\tFF\tFF\tFF\tFF\tFF\t9F\r\n      2345  0CF104A7   00000004    8        F0\t60\t22\tFC\tFF\tFF\tFF\t4F\r\n      2344  0CF103A7   00000004    8        17\t1F\t08\t60\tB1\t1F\t08\t4F\r\n      2344  0CF102A7   00000004    8        30\t75\tE0\t2E\t80\tFF\tFF\tFD\r\n      2343  0C3C4D4A   00000004    8        BE\tFF\tFF\t7F\t18\tFF\tFF\t4F\r\n      2343  0CF101A7   00000004    8        68\t00\t97\tCC\t00\t16\t39\t8F\r\n      2342  18F120F0   00000004    8        2B\t75\t60\tB1\tB0\t01\tFF\tFF\r\n      2363  0CF101A7   00000004    8        68\t00\t97\tCC\t00\t16\t39\t90\r\n      2362  1FFFFFFF   00000004    8        00\t00\tFF\tFF\tFF\tFF\tFF\tFF\r\n      2352  1FFFFFFF   00000004    8        00\t20\tFF\tFF\tFF\tFF\tFF\tFF\r\n      2347  1FFFFFFF   00000004    8        00\t20\tFF\tFF\tFF\tFF\tFF\tFF\r\n      2346  18F121F0   00000004    8        09\t19\t00\t00\tFF\tFF\tB0\t01\r\n      2345  18F106A7   00000004    8        00\tF7\tFF\tFF\tFF\tFF\tFF\t9F\r\n      2345  0CF104A7   00000004    8        F0\t60\t22\tFC\tFF\tFF\tFF\t4F\r\n      2344  0CF103A7   00000004    8        17\t1F\t08\t60\tB1\t1F\t08\t4F\r\n      2344  0CF102A7   00000004    8        30\t75\tE0\t2E\t80\tFF\tFF\tFD\r\n      2343  0C3C4D4A   00000004    8        BE\tFF\tFF\t7F\t18\tFF\tFF\t4F\r\n      2343  0CF101A7   00000004    8        68\t00\t97\tCC\t00\t16\t39\t8F\r\n      2363  0CF102A7   00000004    8        30\t75\tE0\t2E\t80\tFF\tFF\tFD\r\n      2363  0CF101A7   00000004    8        68\t00\t97\tCC\t00\t16\t39\t90\r\n      2362  1FFFFFFF   00000004    8        00\t00\tFF\tFF\tFF\tFF\tFF\tFF\r\n      2352  1FFFFFFF   00000004    8        00\t20\tFF\tFF\tFF\tFF\tFF\tFF\r\n      2347  1FFFFFFF   00000004    8        00\t20\tFF\tFF\tFF\tFF\tFF\tFF\r\n      2346  18F121F0   00000004    8        09\t19\t00\t00\tFF\tFF\tB0\t01\r\n      2345  18F106A7   00000004    8        00\tF7\tFF\tFF\tFF\tFF\tFF\t9F\r\n      2345  0CF104A7   00000004    8        F0\t60\t22\tFC\tFF\tFF\tFF\t4F\r\n      2344  0CF103A7   00000004    8        17\t1F\t08\t60\tB1\t1F\t08\t4F\r\n      2344  0CF102A7   00000004    8        30\t75\tE0\t2E\t80\tFF\tFF\tFD\r\n      2343  0C3C4D4A   00000004    8        BE\tFF\tFF\t7F\t18\tFF\tFF\t4F\r\n      2372  1FFFFFFF   00000004    8        00\t20\tFF\tFF\tFF\tFF\tFF\tFF\r\n      2363  0CF102A7   00000004    8        30\t75\tE0\t2E\t80\tFF\tFF\tFD\r\n      2363  0CF101A7   00000004    8        68\t00\t97\tCC\t00\t16\t39\t90\r\n      2362  1FFFFFFF   00000004    8        00\t00\tFF\tFF\tFF\tFF\tFF\tFF\r\n      2352  1FFFFFFF   00000004    8        00\t20\tFF\tFF\tFF\tFF\tFF\tFF\r\n      2347  1FFFFFFF   00000004    8        00\t20\tFF\tFF\tFF\tFF\tFF\tFF\r\n      2346  18F121F0   00000004    8        09\t19\t00\t00\tFF\tFF\tB0\t01\r\n      2345  18F106A7   00000004    8        00\tF7\tFF\tFF\tFF\tFF\tFF\t9F\r\n      2345  0CF104A7   00000004    8        F0\t60\t22\tFC\tFF\tFF\tFF\t4F\r\n      2344  0CF103A7   00000004    8        17\t1F\t08\t60\tB1\t1F\t08\t4F\r\n      2344  0CF102A7   00000004    8        30\t75
